vi "echo-show-frames.vi"() -> ()   [LabVIEW 2021]
panel:
  in  "show frame":i64(slide)=50000 scale=0.0..100.0
  in  "#of  frames":i64=50000
  out "Numeric":i32
  in  "String":string="D:\\data\\pulsed-echo-brad-Mar2022\\220308_175815000.dat"
  out "XY Graph":cluster{dbl[], dbl[]}(graph)
  in  "File Path":path=path "D:/data/pulsed-echo-brad-Mar2022/220308_175815000.dat"
  out "load":bool
  in  "#of samples per frame":i64=50000
  in  "dt":dbl=4e-11
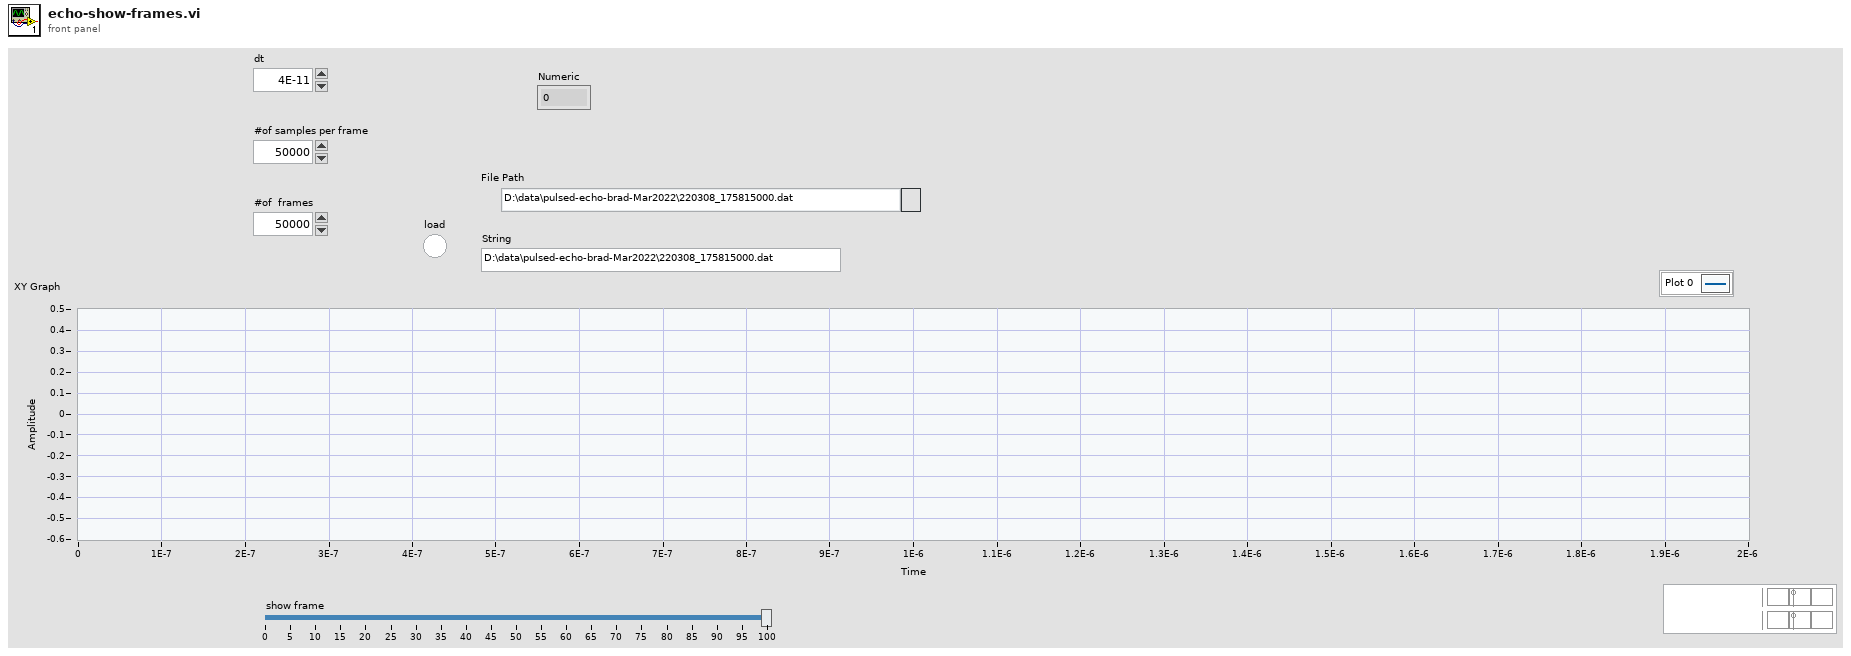
[diagram p1: front panel]
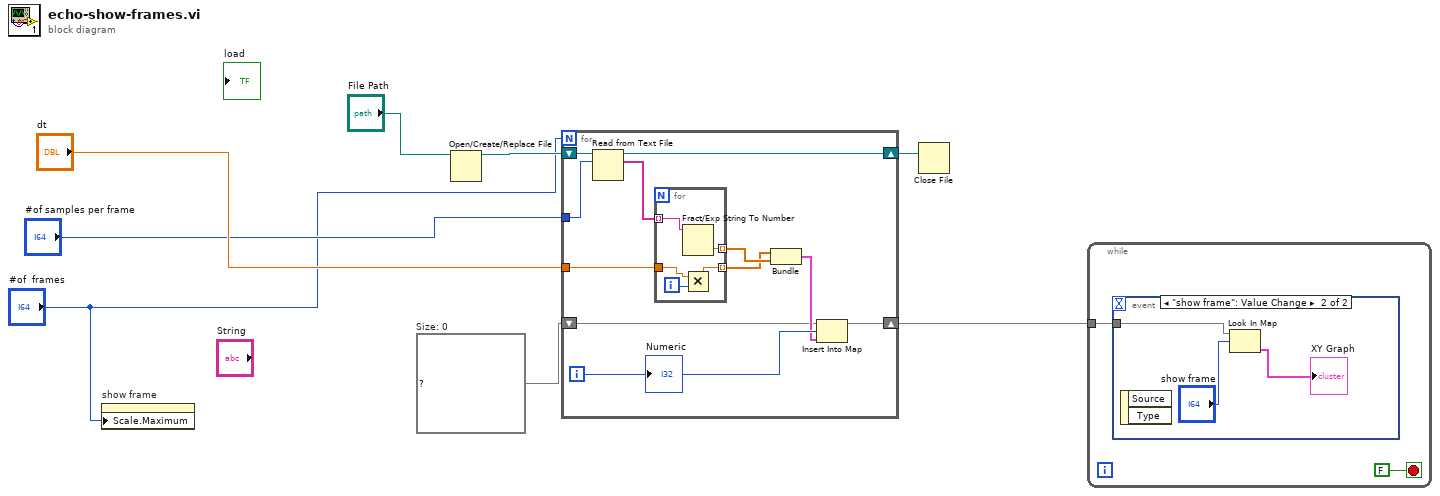
[diagram p0: block diagram]
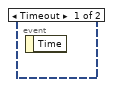
[diagram p2: hidden frame]
diagram:
  w3 = map{i32, cluster{dbl[], dbl[]}} {}  # Size: 0
  n1 = property on="show frame" class="Slide (strict)"("Scale.Maximum"="#of  frames") -> ()  [unwired: 2 in, 2 out]
  n2 = Open/Create/Replace File(file path (use dialog)="File Path") -> (refnum out=w6:refnum<file>)  [unwired: 5 in, 2 out]
  n3 = for {
    N: "#of  frames" -> [_]
    tunnel: "dt" -> [w19]
    tunnel: "#of samples per frame" -> [w18]
    shift-right: [w11] -> w5
    shift-left: w6 -> [w17]
    shift-right: [w13] -> w4
    shift-left: w3 -> [w12]
    i -> [w15]
    n4 = Read from Text File(file (use dialog)=w17, count=w18) -> (refnum out=w11:refnum<file>, text=w16:string[])  [unwired: 2 in, 2 out]
    n5 = for {
      tunnel: [w22] -> w10 mode=indexing
      tunnel: w19 -> [w24]
      tunnel: [w23] -> w9 mode=indexing
      tunnel: w16 -> [w20] mode=indexing
      i -> [w21]
      n6 = Fract/Exp String To Number(string=w20) -> (number=w22:dbl)  [unwired: 3 in, 1 out]
      n7 = Multiply(x=w24, y=w21) -> (x*y=w23:dbl)
    }
    n8 = Bundle(w9, w10) -> (w14:cluster{dbl[], dbl[]})  [unwired: 1 in]
    n9 = Insert Into Map(map in=w12, key=w15, value=w14) -> (map out=w13:map{i32, cluster{dbl[], dbl[]}})  [unwired: 2 out]
    "Numeric" <- w15
  }
  n10 = Close File(refnum=w5) -> ()  [unwired: 1 in, 2 out]
  n11 = while {
    tunnel: w4 -> [w26]
    stop <- FALSE stop-if-true
    n12 = event shown="[1] \"show frame\": Value Change" {
      selector: _ -> [_ _]
      dyn-events: _ -> [_ _]
      timeout: _ -> [_ _]
      tunnel: w26 -> [_ w29]
      event Timeout {
        n13 = event-data() -> ()  [unwired: 1 in, 1 out]
      }
      event "show frame": Value Change {
        n14 = event-data() -> ()  [unwired: 1 in, 2 out]
        n15 = Look In Map(map=w29, key="show frame") -> (value=→"XY Graph":cluster{dbl[], dbl[]})  [unwired: 1 in, 1 out]
      }
    }
  }
